vi "Create Easy Text Report.vi"(0 "text to be printed":string, 1 "margins":T4={"margins (1.00)"={"top"=1.0, "left"=1.0, "right"=1.0, "bottom"=1.0}, "measurement system (default)"=0} {"measurement system (default)" items=["Default", "US", "Metric"]; "margins (1.00)"."right" format="%0.2f"; "margins (1.00)"."bottom" format="%0.2f"; "margins (1.00)"."top" format="%0.2f"; "margins (1.00)"."left" format="%0.2f"}, 2 "print or save?":enum16{"print", "save"}(ring), 3 "font settings":T3={"charset (-1)"=-1, "weight (-1)"=-1, "name"="", "size"=" "}, 5 "printer name (default) or file path (dialog)":string, 7 "report type (HTML)":T1, 9 "orientation (portrait)":i32(ring) items=["portrait", "landscape"], 11 "error in (no error)":errorcluster, 12 "headers":T2, 14 "footers":T2) -> (15 "error out":errorcluster)   [LabVIEW 2020, in "NI_report.lvclass"]
doc: "Allows you to pass in a block of text along with optional formatting information and print the report to a designated printer or publish the report to a specified file path."
uses:
  NI_report.lvclass
  Report Type.ctl
  NI_ReportGenerationCore.lvlib
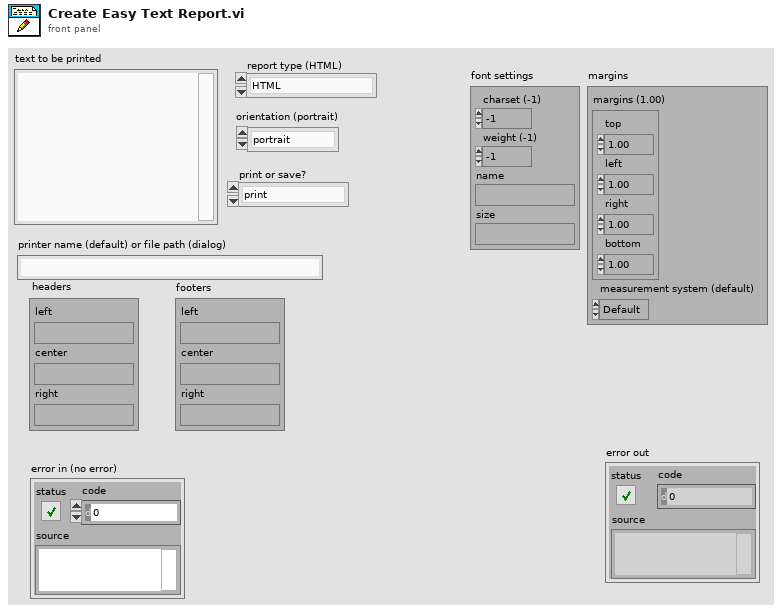
[diagram p1: front panel]
types:
  T1 = typedef "NI_ReportGenerationCore.lvlib/Report Type.ctl" = enum16{"HTML", "Word", "Excel"}
  T2 = cluster{"left":string, "center":string, "right":string}
  T3 = cluster{"charset (-1)":i16, "weight (-1)":i16, "name":string, "size":string}
  T4 = cluster{"margins (1.00)":cluster{"top":dbl, "left":dbl, "right":dbl, "bottom":dbl}, "measurement system (default)":u16}
  T5 = cluster{"top":dbl, "left":dbl, "right":dbl, "bottom":dbl}
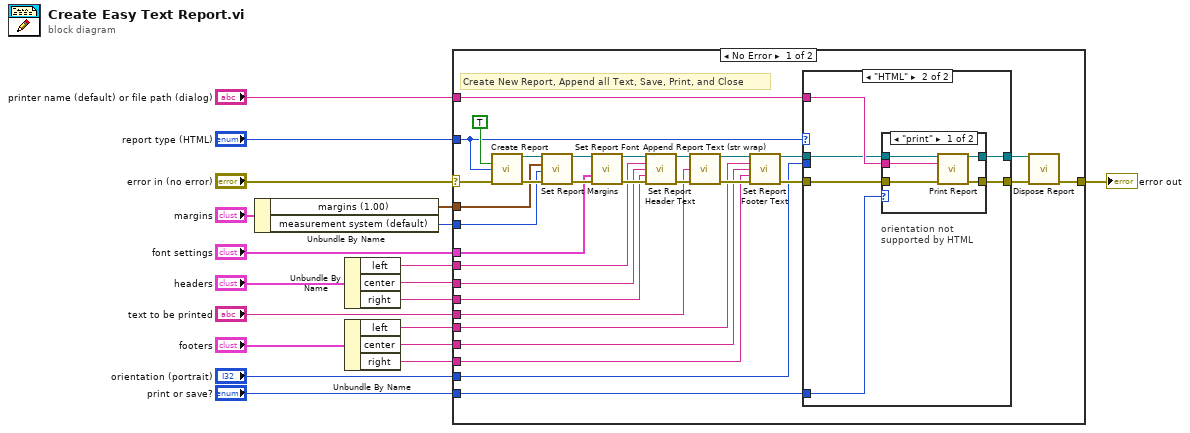
[diagram p0: block diagram]
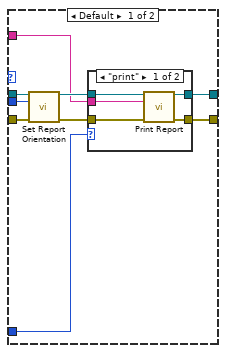
[diagram p2: hidden frame]
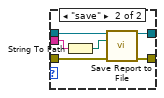
[diagram p3: hidden frame]
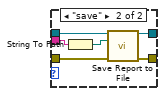
[diagram p4: hidden frame]
diagram:
  n1 = Unbundle By Name("margins") -> ("margins (1.00)"=w17:T5, "measurement system (default)"=w16:u16)
  n2 = Unbundle By Name("headers") -> ("left"=w14:string, "center"=w13:string, "right"=w12:string)
  n3 = Unbundle By Name("footers") -> ("left"=w10:string, "center"=w9:string, "right"=w8:string)
  n4 = case shown="No Error" "error in (no error)" {
    selector: "error in (no error)" -> [w39 w88]
    tunnel: [w40 w88] -> w19
    tunnel: w17 -> [w48 _]
    tunnel: w16 -> [w45 _]
    tunnel: w14 -> [w36 _]
    tunnel: w13 -> [w44 _]
    tunnel: w12 -> [w43 _]
    tunnel: w10 -> [w32 _]
    tunnel: w9 -> [w30 _]
    tunnel: w8 -> [w31 _]
    tunnel: "text to be printed" -> [w29 _]
    tunnel: "orientation (portrait)" -> [w25 _]
    tunnel: "font settings" -> [w28 _]
    tunnel: "report type (HTML)" -> [w24 _]
    tunnel: "printer name (default) or file path (dialog)" -> [w20 _]
    tunnel: "print or save?" -> [w21 _]
    frame No Error {
      # "Create New Report, Append all Text, Save, Print, and Close"
      n5 = call "Create Report.vi"("display alerts? (F)"=TRUE, "report type"=w24, "error in (no error)"=w39) -> ("report out"=w50:refnum<class "NI_report.lvclass">, "error out"=w49:errorcluster)  [unwired: 11 in]
      n6 = call-dynamic "Set Report Margins.vi"("report in"=w50, "margins (1.00)"=w48, "measurement system (default)"=w45, "error in (no error)"=w49) -> ("report out"=w42:refnum<class "NI_report.lvclass">, "error out"=w41:errorcluster)  [unwired: 10 out]
      n7 = call-dynamic "Set Report Font.vi"("report in"=w42, "font settings"=w28, "error in (no error)"=w41) -> ("report out"=w47:refnum<class "NI_report.lvclass">, "error out"=w46:errorcluster)  [unwired: 3 in, 8 out]
      n8 = call-dynamic "Set Report Header Text.vi"("report in"=w47, "left header text"=w36, "center header text"=w44, "right header text"=w43, "error in (no error)"=w46) -> ("report out"=w38:refnum<class "NI_report.lvclass">, "error out"=w33:errorcluster)  [unwired: 2 in, 7 out]
      n9 = call "Append Report Text (str wrap).vi"("report in"=w38, "text"=w29, "error in (no error)"=w33) -> ("report out"=w37:refnum<class "NI_report.lvclass">, "error out"=w34:errorcluster)  [unwired: 9 in, 2 out]
      n10 = call-dynamic "Set Report Footer Text.vi"("report in"=w37, "left footer text"=w32, "center footer text"=w30, "right footer text"=w31, "error in (no error)"=w34) -> ("report out"=w27:refnum<class "NI_report.lvclass">, "error out"=w26:errorcluster)  [unwired: 1 in, 8 out]
      n11 = case shown="\"HTML\"" w24 {
        tunnel: w27 -> [w59 w72]
        tunnel: [w56 w76] -> w23
        tunnel: [w55 w75] -> w22
        tunnel: w26 -> [w58 w71]
        tunnel: w25 -> [w57 _]
        tunnel: w21 -> [w52 w74]
        tunnel: w20 -> [w51 w73]
        frame Default {
          n12 = call-dynamic "Set Report Orientation.vi"("report in"=w59, "orientation (portrait)"=w57, "error in (no error)"=w58) -> ("report out"=w54:refnum<class "NI_report.lvclass">, "error out"=w53:errorcluster)  [unwired: 11 out]
          n13 = case shown="\"print\"" w52 {
            tunnel: w54 -> [w61 w70]
            tunnel: w53 -> [w63 w69]
            tunnel: [w62 w68] -> w56
            tunnel: [w64 w67] -> w55
            tunnel: w51 -> [w60 w66]
            frame "print" {
              n14 = call-dynamic "Print Report.vi"("report in"=w61, "printer name (default)"=w60, "error in (no error)"=w63) -> ("report out"=w62:refnum<class "NI_report.lvclass">, "error out"=w64:errorcluster)  [unwired: 1 in, 10 out]
            }
            frame "save" {
              n15 = String To Path(string=w66) -> (path=w65:path)
              n16 = call-dynamic "Save Report to File.vi"("report in"=w70, "report file path"=w65, "error in (no error)"=w69) -> ("report out"=w68:refnum<class "NI_report.lvclass">, "error out"=w67:errorcluster)  [unwired: 2 in, 9 out]
            }
          }
        }
        frame "HTML" {
          # "orientation not supported by HTML"
          n17 = case shown="\"print\"" w74 {
            tunnel: w72 -> [w78 w87]
            tunnel: w71 -> [w80 w86]
            tunnel: [w79 w85] -> w76
            tunnel: [w81 w84] -> w75
            tunnel: w73 -> [w77 w83]
            frame "print" {
              n18 = call-dynamic "Print Report.vi"("report in"=w78, "printer name (default)"=w77, "error in (no error)"=w80) -> ("report out"=w79:refnum<class "NI_report.lvclass">, "error out"=w81:errorcluster)  [unwired: 1 in, 10 out]
            }
            frame "save" {
              n19 = String To Path(string=w83) -> (path=w82:path)
              n20 = call-dynamic "Save Report to File.vi"("report in"=w87, "report file path"=w82, "error in (no error)"=w86) -> ("report out"=w85:refnum<class "NI_report.lvclass">, "error out"=w84:errorcluster)  [unwired: 2 in, 9 out]
            }
          }
        }
      }
      n21 = call-dynamic "Dispose Report.vi"("report in"=w23, "error in (no error)"=w22) -> ("error out"=w40:errorcluster)  [unwired: 3 in, 10 out]
    }
    frame Error {
    }
  }
  "error out" <- w19
